vi "PH_ImageStatistician.get i attribute.vi"(0 "i ref in":refnum<vi>, 5 "error in (no error)":errorcluster) -> (14 "i ref out":refnum<vi>, 16 "i attribute":T1 {"Data 3" items=["nothing ", "FWHM Major Trace", "FWHM Minor Trace", "Gaussian Fit Order Major Trace", "Gaussian Fit Order Minor Trace", "99% Diameter Major Trace", "99% Diameter Minor Trace", "Theta", "Delta", "Major Diameter", "Minor Diameter", "Azimuth Angle", "Azi Angle rel to Major?", "Ellipticity", "Center of gravity - x", "Center of gravity - y", "Energy"]; "Data 2" items=["nothing ", "FWHM Major Trace", "FWHM Minor Trace", "Gaussian Fit Order Major Trace", "Gaussian Fit Order Minor Trace", "99% Diameter Major Trace", "99% Diameter Minor Trace", "Theta", "Delta", "Major Diameter", "Minor Diameter", "Azimuth Angle", "Azi Angle rel to Major?", "Ellipticity", "Center of gravity - x", "Center of gravity - y", "Energy"]; "Data 1" items=["nothing ", "FWHM Major Trace", "FWHM Minor Trace", "Gaussian Fit Order Major Trace", "Gaussian Fit Order Minor Trace", "99% Diameter Major Trace", "99% Diameter Minor Trace", "Theta", "Delta", "Major Diameter", "Minor Diameter", "Azimuth Angle", "Azi Angle rel to Major?", "Ellipticity", "Center of gravity - x", "Center of gravity - y", "Energy"]}, 19 "error out":errorcluster)   [LabVIEW 2014, in "PH_ImageStatistician.lvlib"]
doc: "Gets the i attribute data of an object.\n\nLicense Agreement for this software:\n\nCopyright (C)\nGesellschaft für Schwerionenforschung, GSI\nPlanckstr. 1\n64291 Darmstadt\nGermany\n\nContact: D.Beck@gsi.de \n\nThis program is free software; you can redistribute it and/or modify it under the terms of the GNU General Public License as published by the Free Software Foundation; either version 2 of the license, or (at your option) any later version.\n\nThis program is distributed in the hope that it will be useful, but WITHOUT ANY WARRANTY; without even the implied warranty of MERCHANTABILITY or FITNESS FOR A PARTICULAR PURPOSE. See the GNU General License for more details (http://www.gnu.org).\n\nGesellschaft für Schwerionenforschung, GSI\nPlanckstr. 1, 64291 Darmstadt, Germany\nFor all questions and ideas contact: M.Richter@gsi.de, H.Brand@gsi.de or D.Beck@gsi.de.\nLast update: 17-JUN-2004"
uses:
  PH_ImageStatistician.lvlib
  PH_ImageStatistician.i attribute.ctl
  PH_ImageStatistician.Statistician Data.ctl
  PH_ImageStatistician.select Data.ctl
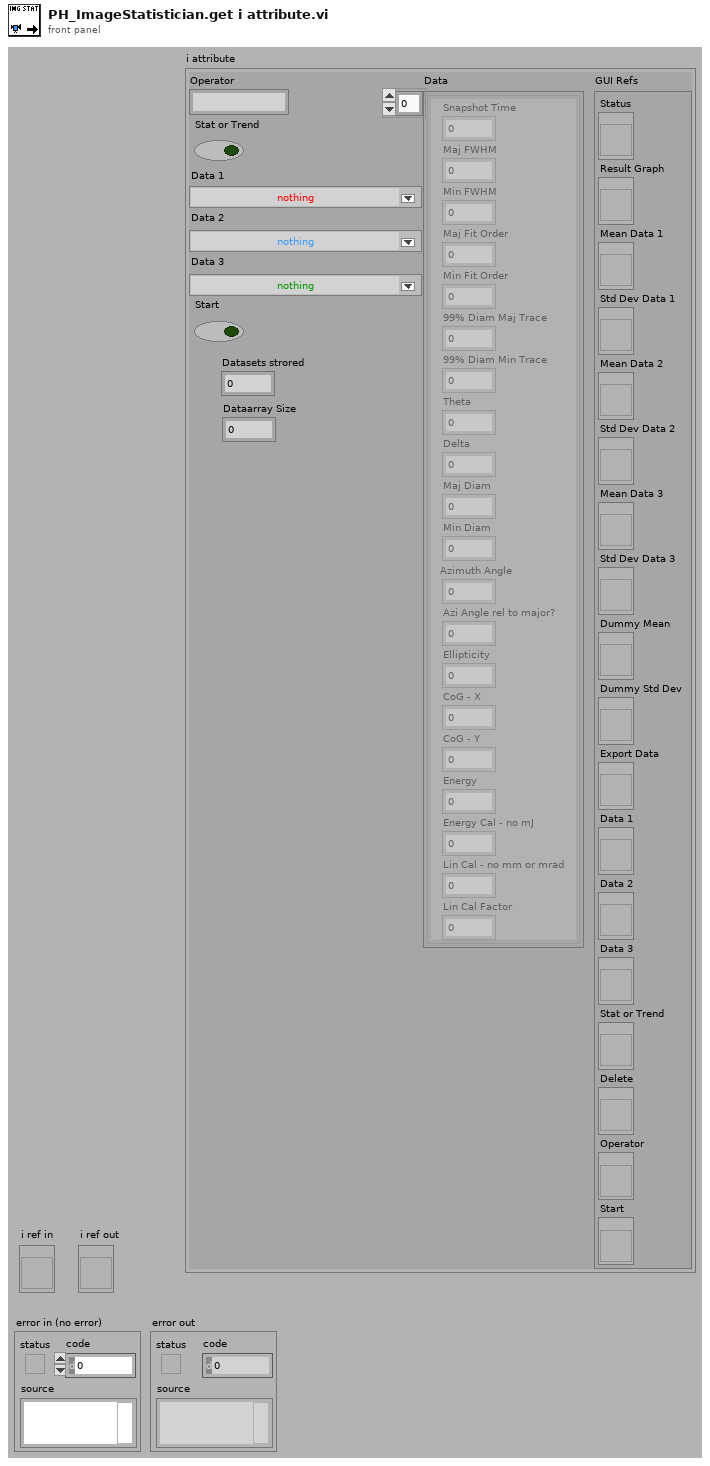
[diagram p1: front panel]
types:
  T1 = typedef "PH_ImageStatistician.lvlib/PH_ImageStatistician.i attribute.ctl" = cluster{"GUI Refs ":cluster{"Status":refnum<vi>, "Result Graph":refnum<vi>, "Mean Data 1":refnum<vi>, "Std Dev Data 1":refnum<vi>, "Mean Data 2":refnum<vi>, "Std Dev Data 2":refnum<vi>, "Mean Data 3":refnum<vi>, "Std Dev Data 3":refnum<vi>, "Dummy Mean":refnum<vi>, "Dummy Std Dev":refnum<vi>, "Export Data":refnum<vi>, "Data 1":refnum<vi>, "Data 2":refnum<vi>, "Data 3":refnum<vi>, "Stat or Trend":refnum<vi>, "Delete":refnum<vi>, "Operator":refnum<vi>, "Start":refnum<vi>}, "Operator":string, "Data":T2[], "Stat or Trend":bool, "Data 1":T3, "Data 2":T3, "Data 3":T3, "Start":bool, "Datasets strored":i32, "Dataarray Size":i32}
  T2 = typedef "PH_ImageStatistician.lvlib/PH_ImageStatistician.Statistician Data.ctl" = cluster{"Snapshot Time":dbl, "Maj FWHM":dbl, "Min FWHM":dbl, "Maj Fit Order":dbl, "Min Fit Order":dbl, "99% Diam Maj Trace":dbl, "99% Diam Min Trace":dbl, "Theta":dbl, "Delta":dbl, "Maj Diam":dbl, "Min Diam":dbl, "Azimuth Angle":dbl, "Azi Angle rel to major?":dbl, "Ellipticity":dbl, "CoG - X":dbl, "CoG - Y":dbl, "Energy":dbl, "Energy Cal - no mJ":dbl, "Lin Cal - no mm or mrad":dbl, "Lin Cal Factor":dbl}
  T3 = typedef "PH_ImageStatistician.lvlib/PH_ImageStatistician.select Data.ctl" = u16
  T4 = enum16{"SetAttribute", "GetAttribute", "CreateAttribute", "DestroyAttribute", "DestroyAllAtributes"}
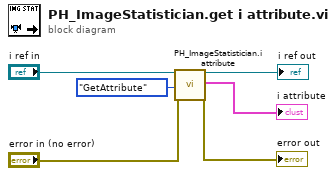
[diagram p0: block diagram]
diagram:
  n1 = call "PH_ImageStatistician.i attribute.vi"("VI Refnum"="i ref in", "Action"=T4."GetAttribute", "error in (no error)"="error in (no error)") -> ("VI Refnum out"=→"i ref out":refnum<vi>, "CLASS.i attribute out"=→"i attribute":T1, "error out"=→"error out":errorcluster)  [unwired: 14 in]
